vi "Send Direct Command.vi"(0 "Dynamixel Motor VISA in":refnum<class "Dynamixel Motor VISA.lvclass">, 5 "Motor ID (0)":u8, 7 "Address":u8, 9 "Select Action":u16(ring) items=["Ping", "Read", "Write", "Registered Write", "Action", "Reset", "Sync Write"], 11 "error in (no error)":errorcluster, 12 "Parameters":string) -> (4 "Dynamixel Motor VISA out":refnum<class "Dynamixel Motor VISA.lvclass">, 6 "Command to Serial":string, 15 "error out":errorcluster)   [LabVIEW 2016, in "Dynamixel Motor VISA.lvclass"]
doc: "Using any of the six basic commands for the Dynamixel motor, this VI allows you to send any set of parameters to the motor(s). This is a Low-Level VI that is used by other VIs."
uses:
  <instrlib>/Dynamixel Motor/HAIOL/VISA/Dynamixel Motor VISA.lvclass
  <instrlib>/Dynamixel Motor/HAIOL/VISA/Dynamixel Motor VISA.lvclass/Dynamixel Motor VISA.ctl
  <instrlib>/Dynamixel Motor/Dynamixel Motor.lvlib
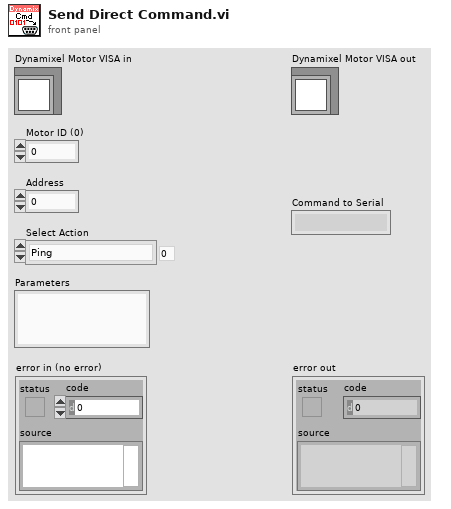
[diagram p1: front panel]
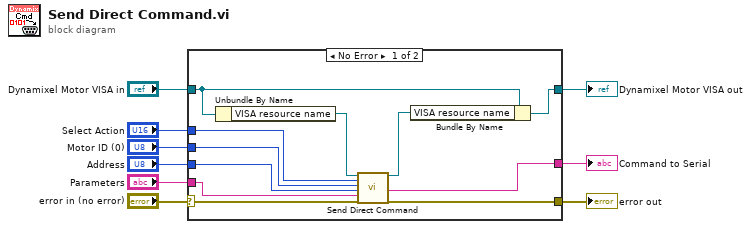
[diagram p0: block diagram]
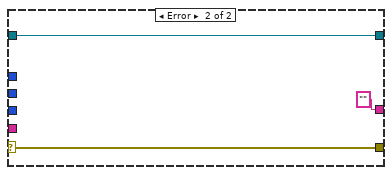
[diagram p2: hidden frame]
diagram:
  n1 = case shown="No Error" "error in (no error)" {
    selector: "error in (no error)" -> [w20 w23]
    tunnel: "Dynamixel Motor VISA in" -> [w12 w21]
    tunnel: "Select Action" -> [w18 _]
    tunnel: "Motor ID (0)" -> [w17 _]
    tunnel: "Address" -> [w16 _]
    tunnel: "Parameters" -> [w15 _]
    tunnel: [w14 w23] -> w3
    tunnel: [w11 w21] -> w2
    tunnel: [w10 "" ("Command to Serial")] -> w1
    frame No Error {
      n2 = Unbundle By Name(w12) -> ("VISA resource name"=w19:refnum<visa-resource-name>)
      n3 = call <instrlib>:"Send Direct Command.vi"("VISA resource name"=w19, "Select Action"=w18, "Motor ID (0)"=w17, "Address"=w16, "Parameters"=w15, "Error in (no error)"=w20) -> ("VISA resource name out"=w13:refnum<visa-resource-name>, "Command to Serial"=w10:string, "Error out"=w14:errorcluster)  [unwired: 11 in]
      n4 = Bundle By Name(cluster=w12, "VISA resource name"=w13) -> (w11:refnum<class "Dynamixel Motor VISA.lvclass">)
    }
    frame Error {
    }
  }
  "error out" <- w3
  "Dynamixel Motor VISA out" <- w2
  "Command to Serial" <- w1
